vi "FGV_timing.vi"(7 "Enum":T1, 8 "error in (no error)":errorcluster, 11 "Target time":dbl) -> (0 "error out":errorcluster, 1 "Elapsed?":bool, 3 "Elapsed Time":dbl)   [LabVIEW 2013]
uses:
  FGV_enum.ctl
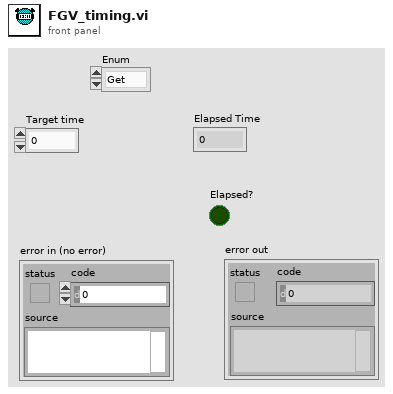
[diagram p1: front panel]
types:
  T1 = typedef "FGV_enum.ctl" = enum16{"Get", "Set"}
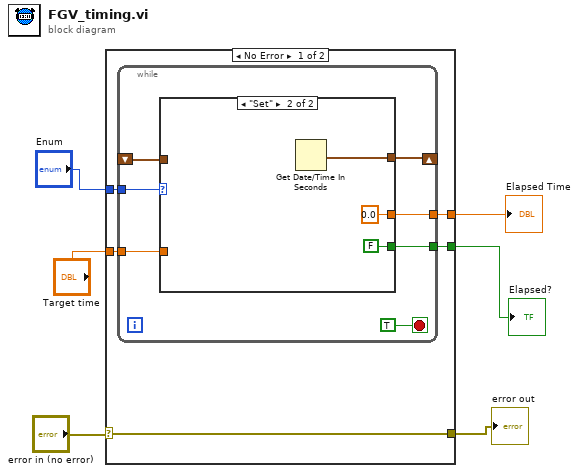
[diagram p0: block diagram]
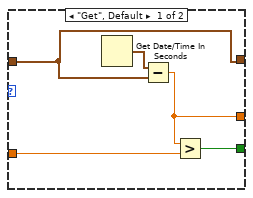
[diagram p2: hidden frame]
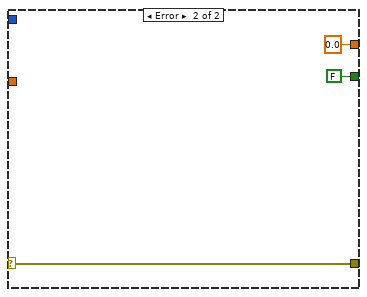
[diagram p3: hidden frame]
diagram:
  n1 = case shown="No Error" "error in (no error)" {
    selector: "error in (no error)" -> [w7 w29]
    tunnel: "Enum" -> [w11 _]
    tunnel: "Target time" -> [w10 _]
    tunnel: [w9 FALSE] -> w4
    tunnel: [w8 0.0] -> w3
    tunnel: [w7 w29] -> w1
    frame No Error {
      n2 = while {
        tunnel: w11 -> [w18]
        shift-right: [w17] -> _
        shift-left: _ -> [w16]
        tunnel: w10 -> [w15]
        tunnel: [w14] -> w9
        tunnel: [w13] -> w8
        stop <- TRUE stop-if-true
        n3 = case shown="\"Set\"" w18 {
          tunnel: [w19 w26] -> w17
          tunnel: w16 -> [w19 _]
          tunnel: w15 -> [w22 _]
          tunnel: [w21 FALSE] -> w14
          tunnel: [w20 0.0] -> w13
          frame "Get", Default {
            n4 = Get Date/Time In Seconds() -> (seconds since 1Jan1904=w23:timestamp)
            n5 = Subtract(x=w23, y=w19) -> (x-y=w20:dbl)
            n6 = Greater?(x=w20, y=w22) -> (0:w21:bool)
          }
          frame "Set" {
            n7 = Get Date/Time In Seconds() -> (seconds since 1Jan1904=w26:timestamp)
          }
        }
      }
    }
    frame Error {
    }
  }
  "Elapsed?" <- w4
  "Elapsed Time" <- w3
  "error out" <- w1
